vi "Read.vi"(8 "error in (no error)":errorcluster, 9 "Trim RX? (T)":bool, 10 "Max bytes to read (999)":u32=999, 11 "Serial Device in":refnum<class "Serial Device.lvclass">) -> (0 "error out":errorcluster, 3 "Serial Device out":refnum<class "Serial Device.lvclass">)   [LabVIEW 2015, in "Serial Device.lvclass"]
uses:
  Serial Device.lvclass
  Serial Device.lvclass/Serial Device.ctl
panel:
  out "RX Data":string
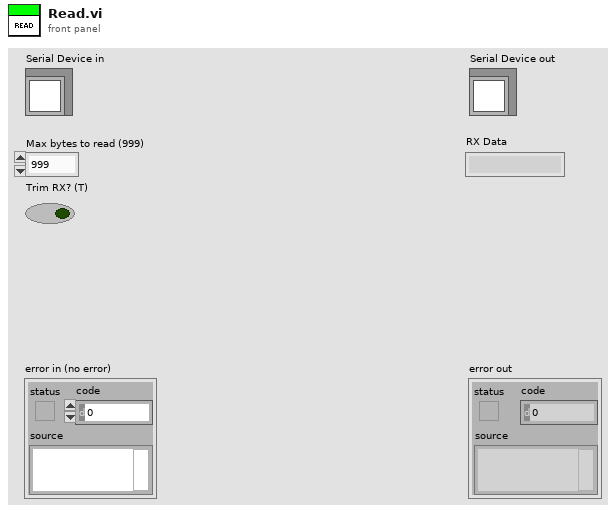
[diagram p1: front panel]
types:
  T1 = typedef "Semaphore RefNum" = refnum<k1>
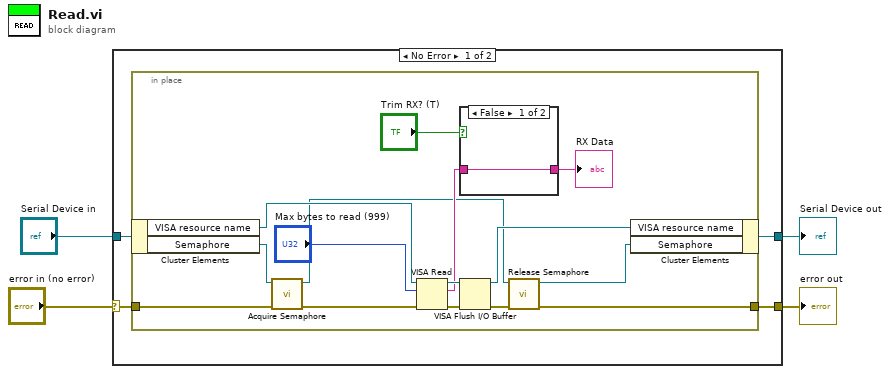
[diagram p0: block diagram]
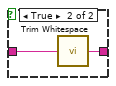
[diagram p2: hidden frame]
diagram:
  n1 = case shown="No Error" "error in (no error)" {
    selector: "error in (no error)" -> [w8 w28]
    tunnel: [w5 w28] -> w3
    tunnel: [w6 w27] -> w1
    tunnel: "Serial Device in" -> [w7 w27]
    frame No Error {
      n2 = in-place {
        in-place-border: w8 -> [w22]
        in-place-border: [w10] -> w5
        n3 = in-place-cluster #1(w7) -> ("VISA resource name"=w20:refnum<visa-resource-name>, "Semaphore"=w19:T1)
        n4 = call <vilib>:"Acquire Semaphore.vi"("error in (no error)"=w22, "semaphore"=w19) -> ("error out"=w21:errorcluster, "semaphore out"=w11:T1)  [unwired: 3 in, 1 out]
        n5 = VISA Read(VISA resource name=w20, byte count="Max bytes to read (999)", error in (no error)=w21) -> (VISA resource name out=w18:refnum<visa-resource-name>, read buffer=w15:string, error out=w13:errorcluster)  [unwired: 1 out]
        n6 = case shown="False" "Trim RX? (T)" {
          tunnel: [w24 w26] -> w16
          tunnel: w15 -> [w24 w25]
          frame False {
          }
          frame True {
            n7 = call <vilib>:"Trim Whitespace.vi"("string"=w25) -> ("trimmed string"=w26:string)  [unwired: 1 in]
          }
        }
        "RX Data" <- w16
        n8 = VISA Flush I/O Buffer(VISA resource name=w18, error in (no error)=w13) -> (VISA resource name out=w17:refnum<visa-resource-name>, error out=w14:errorcluster)  [unwired: 1 in]
        n9 = call <vilib>:"Release Semaphore.vi"("error in (no error)"=w14, "semaphore"=w11) -> ("error out"=w10:errorcluster, "semaphore out"=w12:T1)  [unwired: 4 in]
        n10 = in-place-cluster #1("VISA resource name"=w17, "Semaphore"=w12) -> (w6:refnum<class "Serial Device.lvclass">)
      }
    }
    frame Error {
    }
  }
  "error out" <- w3
  "Serial Device out" <- w1
